vi "Run.vi"(7 "Data":refnum<class "Datum.lvclass">, 8 "Error In":errorcluster, 11 "Compiler In":refnum<class "Compiler.lvclass">) -> (0 "Error Out":errorcluster, 3 "Compiler Out":refnum<class "Compiler.lvclass">)   [LabVIEW 2018, in "Toolkit.lvlib" / "Compiler.lvclass"]
uses:
  Compiler.lvclass
  Data/Datum/Datum.lvclass
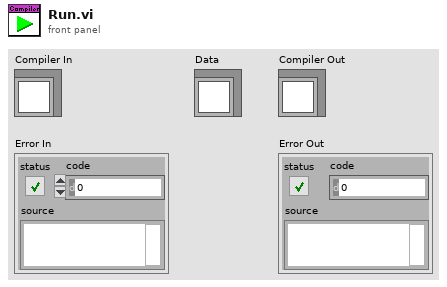
[diagram p1: front panel]
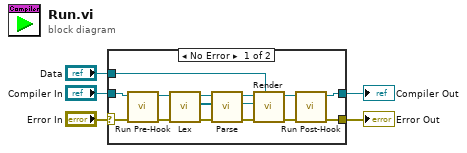
[diagram p0: block diagram]
diagram:
  n1 = case shown="No Error" "Error In" {
    selector: "Error In" -> [w17 w21]
    tunnel: "Compiler In" -> [w18 w22]
    tunnel: [w16 w22] -> w3
    tunnel: [w15 w21] -> w2
    tunnel: "Data" -> [w6 _]
    frame No Error {
      n2 = call-dynamic "Run Pre-Hook.vi"("Error In"=w17, "Compiler In"=w18) -> ("Error Out"=w19:errorcluster, "Compiler Out"=w20:refnum<class "Compiler.lvclass">)  [unwired: 8 in]
      n3 = call-dynamic "Lex.vi"("Error In"=w19, "Compiler In"=w20) -> ("Error Out"=w13:errorcluster, "Tokens"=w12:refnum<class "Token.lvclass">[], "Compiler Out"=w14:refnum<class "Compiler.lvclass">)  [unwired: 7 in]
      n4 = call-dynamic "Parse.vi"("Error In"=w13, "Tokens"=w12, "Compiler In"=w14) -> ("Error Out"=w7:errorcluster, "Abstract Syntax Tree"=w9:refnum<class "Root.lvclass">, "Compiler Out"=w11:refnum<class "Compiler.lvclass">)  [unwired: 6 in]
      n5 = call "Render.vi"("Data"=w6, "Error In"=w7, "Abstract Syntax Tree"=w9, "Compiler In"=w11) -> ("Error Out"=w8:errorcluster, "Compiler Out"=w10:refnum<class "Compiler.lvclass">)  [unwired: 6 in]
      n6 = call-dynamic "Run Post-Hook.vi"("Error In"=w8, "Compiler In"=w10) -> ("Error Out"=w15:errorcluster, "Compiler Out"=w16:refnum<class "Compiler.lvclass">)  [unwired: 8 in]
    }
    frame Error {
    }
  }
  "Compiler Out" <- w3
  "Error Out" <- w2
